vi "Read PID Components.vi"(0 "VISA resource name":refnum<visa-resource-name>, 1 "Unit Address (1)":u8=1 min=1 max=254, 11 "error in (no error)":errorcluster) -> (3 "Derivative Component of\nOutput":sgl, 4 "VISA resource name out":refnum<visa-resource-name>, 6 "Proportional Band":sgl, 10 "Integral Component of\nOutput":sgl, 15 "error out":errorcluster)   [LabVIEW 2010, in "Eurotherm 32xx Series.lvlib"]
doc: "This VI returns Components of Output."
uses:
  <instrlib>/Eurotherm 32xx Series/Eurotherm 32xx Series.lvlib
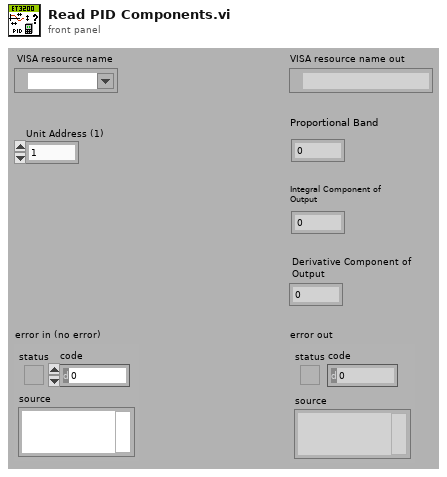
[diagram p1: front panel]
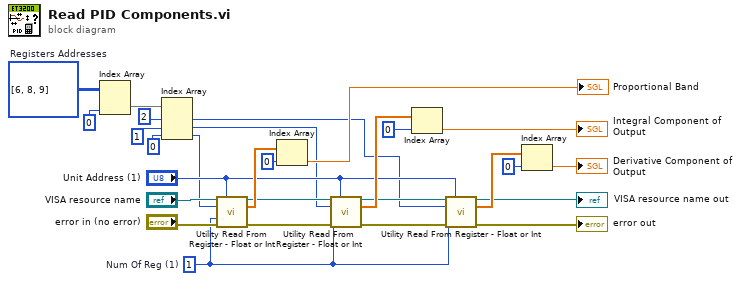
[diagram p0: block diagram]
diagram:
  w9 = u16[][] [[6], [8], [9]]  # Registers Addresses
  w13 = u16 1  # Num Of Reg (1)
  n1 = Index Array(array=w9, index (col)=0 ("Number of PID (1)")) -> (element=w8:u16[])  [unwired: 1 in]
  n2 = Index Array(array=w8, index #1=2 ("index"), index #2=1 ("index"), index #3=0 ("index")) -> (element #1=w2:u16, element #2=w3:u16, element #3=w4:u16)
  n3 = call <instrlib>:"Utility Read From Register - Float or Int.vi"("VISA resource name"="VISA resource name", "Unit Address (1)"="Unit Address (1)", "Register Address (0)"=w4, "Num Of Reg (1)"=w13, "error in (no error)"="error in (no error)") -> ("VISA resource name out"=w23:refnum<visa-resource-name>, "Data"=w26:sgl[], "error out"=w22:errorcluster)  [unwired: 8 in]
  n4 = Index Array(array=w26, index=0) -> (element=→"Proportional Band":sgl)
  n5 = call <instrlib>:"Utility Read From Register - Float or Int.vi"("VISA resource name"=w23, "Unit Address (1)"="Unit Address (1)", "Register Address (0)"=w3, "Num Of Reg (1)"=w13, "error in (no error)"=w22) -> ("VISA resource name out"=w16:refnum<visa-resource-name>, "Data"=w20:sgl[], "error out"=w15:errorcluster)  [unwired: 8 in]
  n6 = Index Array(array=w20, index=0) -> (element=→"Integral Component of\nOutput":sgl)
  n7 = call <instrlib>:"Utility Read From Register - Float or Int.vi"("VISA resource name"=w16, "Unit Address (1)"="Unit Address (1)", "Register Address (0)"=w2, "Num Of Reg (1)"=w13, "error in (no error)"=w15) -> ("VISA resource name out"=→"VISA resource name out":refnum<visa-resource-name>, "Data"=w18:sgl[], "error out"=→"error out":errorcluster)  [unwired: 8 in]
  n8 = Index Array(array=w18, index=0) -> (element=→"Derivative Component of\nOutput":sgl)
